vi "boolean to temperature.vi"(11 "SPI array":u8[](array[numeric])) -> (3 "Temperatura":dbl)   [LabVIEW 2021]
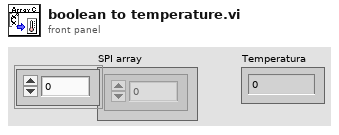
[diagram p1: front panel]
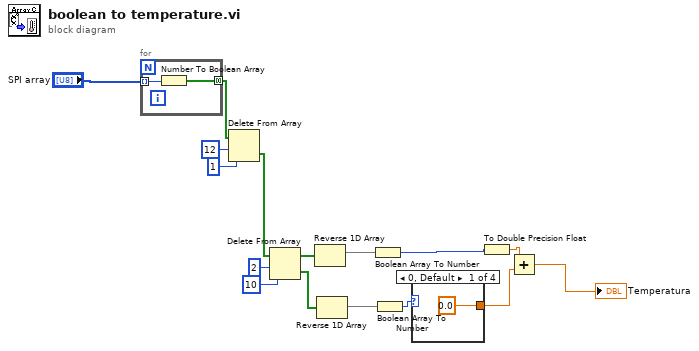
[diagram p0: block diagram]
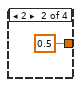
[diagram p2: hidden frame]
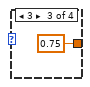
[diagram p3: hidden frame]
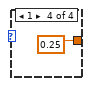
[diagram p4: hidden frame]
diagram:
  n1 = for {
    tunnel: "SPI array" -> [w18] mode=indexing
    tunnel: [w17] -> w1 mode=concatenating
    n2 = Number To Boolean Array(number=w18) -> (Boolean array=w17:bool[])
  }
  n3 = Delete From Array(array=w1, length=12, index=1) -> (deleted portion=w4:bool[])  [unwired: 1 out]
  n4 = Delete From Array(array=w4, length=2, index=10) -> (deleted portion=w8:bool[], array with subset deleted=w7:bool[])
  n5 = Reverse 1D Array(array=w7) -> (reversed array=w9:bool[])
  n6 = Reverse 1D Array(array=w8) -> (reversed array=w10:bool[])
  n7 = Boolean Array To Number(Boolean array=w9) -> (number=w12:u32)
  n8 = Boolean Array To Number(Boolean array=w10) -> (number=w11:u32)
  n9 = case shown="0, Default" w11 {
    tunnel: [0.0 0.5 0.75 0.25] -> w14
    frame 0, Default {
    }
    frame 2 {
    }
    frame 3 {
    }
    frame 1 {
    }
  }
  n10 = To Double Precision Float(number=w12) -> (double precision float=w13:dbl)
  n11 = Add(x=w13, y=w14) -> (x+y=→"Temperatura":dbl)
